vi "Puzzle 1-1.vi"() -> ()   [LabVIEW 2022 SP3]
panel:
  out "sum":i32=54450
  out "Array 3":i32[](array[numeric])=[11, 53, 81, 79, 28, 61, 81, 25, 44, 61, 17, 88, 22, 94, 45, 76, 32, 22, 13, 88, 17, 66, 11, 75, 55, 22, 75, 77, 79, 45, 55, 81, 33, 89, 76, 24, 73, 86, 22, 71, 99, 15, 66, 11, 11, 26, 99, 97, 77, 82, 33, 52, 95, 44, 22, 28, 34, 44, 28, 18, 77, 61, 86, 32, 66, 99, 66, 32, 91, 55, 43, 44, 12, 41, 96, 25, 77, 11, 27, 87, 88, 43, 16, 27, 55, 44, 22, 55, 71, 97, 83, 79, 99, 62, 27, 11, 88, 11, 66, 45, 63, 53, 33, 41, 35, 53, 92, 44, 22, 19, 65, 44, 11, 78, 58, 13, 13, 47, 11, 77, 55, 66, 32, 22, 11, 22, 54, 44, 96, 13, 59, 71, 22, 88, 29, 58, 33, 98, 43, 65, 11, 44, 66, 33, 74, 58, 41, 66, 38, 11, 81, 44, 99, 99, 83, 99, 33, 67, 75, 33, 75, 33, 55, 22, 88, 22, 29, 69, 33, 18, 39, 11, 36, 22, 98, 34, 32, 54, 48, 71, 56, 88, 51, 18, 11, 71, 77, 33, 55, 77, 21, 16, 14, 21, 16, 69, 88, 49, 31, 98, 85, 33, 14, 66, 62, 91, 88, 62, 68, 22, 14, 24, 94, 62, 58, 62, 19, 41, 67, 61, 59, 77, 92, 38, 77, 72, 95, 77, 35, 45, 33, 89, 77, 77, 31, 13, 46, 48, 77, 33, 71, 55, 85, 11, 63, 77, 55, 83, 88, 87, 44, 34, 33, 97, 55, 99, 55, 77, 27, 21, 22, 66, 55, 28, 42, 33, 84, 82, 64, 21, 78, 55, 58, 82, 34, 13, 62, 53, 28, 22, 94, 22, 85, 88, 47, 31, 88, 32, 33, 77, 47, 57, 21, 17, 54, 77, 32, 11, 66, 71, 93, 33, 49, 66, 11, 83, 23, 99, 27, 11, 85, 95, 85, 46, 12, 38, 86, 13, 52, 66, 78, 82, 77, 77, 11, 44, 99, 89, 88, 31, 55, 44, 42, 75, 66, 42, 19, 88, 58, 78, 77, 32, 15, 44, 77, 76, 85, 28, 93, 37, 42, 22, 11, 14, 22, 82, 86, 77, 93, 99, 44, 54, 99, 22, 88, 55, 17, 11, 61, 13, 57, 39, 66, 55, 27, 94, 41, 49, 66, 61, 11, 22, 99, 27, 55, 24, 34, 73, 95, 72, 59, 88, 24, 24, 98, 63, 29, 77, 55, 39, 99, 89, 16, 38, 92, 37, 98, 66, 99, 57, 27, 23, 44, 47, 88, 79, 33, 55, 88, 11, 99, 77, 32, 66, 77, 64, 57, 99, 69, 44, 63, 56, 55, 99, 33, 66, 44, 17, 43, 98, 74, 24, 11, 93, 33, 23, 41, 99, 74, 64, 85, 91, 57, 77, 88, 79, 49, 33, 44, 33, 91, 29, 17, 51, 64, 82, 75, 53, 11, 21, 51, 33, 46, 91, 55, 22, 98, 59, 66, 66, 44, 14, 55, 44, 61, 29, 39, 91, 66, 76, 78, 97, 52, 44, 53, 17, 35, 26, 33, 55, 44, 77, 24, 97, 44, 33, 94, 43, 99, 47, 24, 44, 72, 63, 44, 72, 12, 55, 88, 42, 28, 44, 67, 47, 33, 68, 95, 75, 66, 92, 34, 77, 54, 84, 66, 74, 29, 25, 81, 18, 11, 98, 24, 32, 29, 88, 35, 88, 34, 33, 55, 61, 41, 11, 33, 45, 39, 86, 77, 77, 77, 23, 87, 89, 77, 77, 55, 98, 56, 22, 92, 99, 87, 66, 35, 33, 15, 88, 11, 25, 13, 47, 23, 52, 86, 99, 68, 33, 44, 99, 87, 11, 77, 22, 81, 27, 48, 83, 22, 22, 72, 77, 33, 56, 18, 59, 44, 11, 11, 15, 77, 33, 84, 87, 73, 99, 88, 48, 43, 88, 37, 52, 91, 95, 77, 57, 67, 44, 84, 33, 99, 34, 44, 33, 66, 75, 61, 67, 84, 26, 52, 11, 55, 99, 48, 37, 55, 71, 44, 68, 19, 33, 94, 29, 81, 22, 92, 44, 21, 87, 66, 66, 22, 33, 68, 85, 44, 85, 44, 68, 37, 15, 22, 31, 44, 61, 53, 34, 45, 86, 36, 55, 48, 96, 88, 94, 85, 55, 41, 44, 47, 22, 33, 44, 29, 44, 54, 97, 18, 44, 76, 36, 43, 83, 99, 99, 71, 73, 41, 85, 88, 99, 59, 26, 47, 98, 28, 72, 44, 11, 11, 52, 44, 32, 25, 96, 18, 33, 56, 55, 44, 98, 61, 77, 11, 45, 94, 16, 65, 79, 88, 62, 77, 55, 61, 28, 99, 31, 67, 27, 78, 35, 66, 99, 42, 22, 77, 66, 37, 27, 22, 49, 66, 94, 54, 84, 14, 51, 29, 44, 91, 45, 46, 19, 18, 88, 22, 46, 92, 85, 89, 75, 27, 11, 33, 56, 77, 22, 75, 15, 53, 25, 33, 58, 16, 59, 36, 45, 42, 64, 59, 44, 66, 33, 34, 59, 38, 56, 66, 75, 22, 24, 27, 27, 11, 26, 22, 42, 22, 28, 99, 98, 44, 78, 66, 65, 19, 59, 28, 77, 98, 92, 65, 11, 16, 22, 66, 66, 38, 79, 75, 99, 11, 15, 66, 95, 22, 88, 14, 22, 52, 82, 22, 46, 83, 66, 77, 81, 22, 83, 58, 68, 55, 38, 26, 54, 55, 33, 53, 11, 33, 85, 81, 95, 32, 74, 99, 71, 23, 11, 25, 74, 94, 88, 23, 39, 53, 11, 13, 96, 44, 88, 54, 26, 66, 77, 33, 99, 54, 17, 85, 77, 23, 66, 54, 97, 55, 78, 36, 33, 27, 69, 16, 49, 66, 62, 76, 88, 86, 65, 45, 24, 44, 68, 33, 46, 33, 96, 96, 22, 44, 86, 77, 52, 66, 83, 55, 64, 11, 55, 69, 33, 88, 55, 55, 19, 95, 94, 46, 31, 88, 32, 77, 48, 22, 49, 77, 96, 49, 55, 33, 81, 98, 33, 33, 24, 97, 55, 45, 77, 48, 11, 77, 44, 44, 69, 43, 67, 99, 58, 76, 66, 42, 88, 46, 55, 88, 66, 99, 51, 42, 65, 47, 82, 59, 43, 22, 87, 77, 29]
  out "Array 2":string[](array[string])=["1", "5", "8", "7", "2", "6", "8", "2", "4", "6", "1", "8", "2", "9", "4", "7", "3", "2", "1", "8", "1", "6", "1", "7", "5", "2", "7", "7", "7", "4", "5", "8", "3", "8", "7", "2", "7", "8", "2", "7", "9", "1", "6", "1", "1", "2", "9", "9", "7", "8", "3", "5", "9", "4", "2", "2", "3", "4", "2", "1", "7", "6", "8", "3", "6", "9", "6", "3", "9", "5", "4", "4", "1", "4", "9", "2", "7", "1", "2", "8", "8", "4", "1", "2", "5", "4", "2", "5", "7", "9", "8", "7", "9", "6", "2", "1", "8", "1", "6", "4", "6", "5", "3", "4", "3", "5", "9", "4", "2", "1", "6", "4", "1", "7", "5", "1", "1", "4", "1", "7", "5", "6", "3", "2", "1", "2", "5", "4", "9", "1", "5", "7", "2", "8", "2", "5", "3", "9", "4", "6", "1", "4", "6", "3", "7", "5", "4", "6", "3", "1", "8", "4", "9", "9", "8", "9", "3", "6", "7", "3", "7", "3", "5", "2", "8", "2", "2", "6", "3", "1", "3", "1", "3", "2", "9", "3", "3", "5", "4", "7", "5", "8", "5", "1", "1", "7", "7", "3", "5", "7", "2", "1", "1", "2", "1", "6", "8", "4", "3", "9", "8", "3", "1", "6", "6", "9", "8", "6", "6", "2", "1", "2", "9", "6", "5", "6", "1", "4", "6", "6", "5", "7", "9", "3", "7", "7", "9", "7", "3", "4", "3", "8", "7", "7", "3", "1", "4", "4", "7", "3", "7", "5", "8", "1", "6", "7", "5", "8", "8", "8", "4", "3", "3", "9", "5", "9", "5", "7", "2", "2", "2", "6", "5", "2", "4", "3", "8", "8", "6", "2", "7", "5", "5", "8", "3", "1", "6", "5", "2", "2", "9", "2", "8", "8", "4", "3", "8", "3", "3", "7", "4", "5", "2", "1", "5", "7", "3", "1", "6", "7", "9", "3", "4", "6", "1", "8", "2", "9", "2", "1", "8", "9", "8", "4", "1", "3", "8", "1", "5", "6", "7", "8", "7", "7", "1", "4", "9", "8", "8", "3", "5", "4", "4", "7", "6", "4", "1", "8", "5", "7", "7", "3", "1", "4", "7", "7", "8", "2", "9", "3", "4", "2", "1", "1", "2", "8", "8", "7", "9", "9", "4", "5", "9", "2", "8", "5", "1", "1", "6", "1", "5", "3", "6", "5", "2", "9", "4", "4", "6", "6", "1", "2", "9", "2", "5", "2", "3", "7", "9", "7", "5", "8", "2", "2", "9", "6", "2", "7", "5", "3", "9", "8", "1", "3", "9", "3", "9", "6", "9", "5", "2", "2", "4", "4", "8", "7", "3", "5", "8", "1", "9", "7", "3", "6", "7", "6", "5", "9", "6", "4", "6", "5", "5", "9", "3", "6", "4", "1", "4", "9", "7", "2", "1", "9", "3", "2", "4", "9", "7", "6", "8", "9", "5", "7", "8", "7", "4", "3", "4", "3", "9", "2", "1", "5", "6", "8", "7", "5", "1", "2", "5", "3", "4", "9", "5", "2", "9", "5", "6", "6", "4", "1", "5", "4", "6", "2", "3", "9", "6", "7", "7", "9", "5", "4", "5", "1", "3", "2", "3", "5", "4", "7", "2", "9", "4", "3", "9", "4", "9", "4", "2", "4", "7", "6", "4", "7", "1", "5", "8", "4", "2", "4", "6", "4", "3", "6", "9", "7", "6", "9", "3", "7", "5", "8", "6", "7", "2", "2", "8", "1", "1", "9", "2", "3", "2", "8", "3", "8", "3", "3", "5", "6", "4", "1", "3", "4", "3", "8", "7", "7", "7", "2", "8", "8", "7", "7", "5", "9", "5", "2", "9", "9", "8", "6", "3", "3", "1", "8", "1", "2", "1", "4", "2", "5", "8", "9", "6", "3", "4", "9", "8", "1", "7", "2", "8", "2", "4", "8", "2", "2", "7", "7", "3", "5", "1", "5", "4", "1", "1", "1", "7", "3", "8", "8", "7", "9", "8", "4", "4", "8", "3", "5", "9", "9", "7", "5", "6", "4", "8", "3", "9", "3", "4", "3", "6", "7", "6", "6", "8", "2", "5", "1", "5", "9", "4", "3", "5", "7", "4", "6", "1", "3", "9", "2", "8", "2", "9", "4", "2", "8", "6", "6", "2", "3", "6", "8", "4", "8", "4", "6", "3", "1", "2", "3", "4", "6", "5", "3", "4", "8", "3", "5", "4", "9", "8", "9", "8", "5", "4", "4", "4", "2", "3", "4", "2", "4", "5", "9", "1", "4", "7", "3", "4", "8", "9", "9", "7", "7", "4", "8", "8", "9", "5", "2", "4", "9", "2", "7", "4", "1", "1", "5", "4", "3", "2", "9", "1", "3", "5", "5", "4", "9", "6", "7", "1", "4", "9", "1", "6", "7", "8", "6", "7", "5", "6", "2", "9", "3", "6", "2", "7", "3", "6", "9", "4", "2", "7", "6", "3", "2", "2", "4", "6", "9", "5", "8", "1", "5", "2", "4", "9", "4", "4", "1", "1", "8", "2", "4", "9", "8", "8", "7", "2", "1", "3", "5", "7", "2", "7", "1", "5", "2", "3", "5", "1", "5", "3", "4", "4", "6", "5", "4", "6", "3", "3", "5", "3", "5", "6", "7", "2", "2", "2", "2", "1", "2", "2", "4", "2", "2", "9", "9", "4", "7", "6", "6", "1", "5", "2", "7", "9", "9", "6", "1", "1", "2", "6", "6", "3", "7", "7", "9", "1", "1", "6", "9", "2", "8", "1", "2", "5", "8", "2", "4", "8", "6", "7", "8", "2", "8", "5", "6", "5", "3", "2", "5", "5", "3", "5", "1", "3", "8", "8", "9", "3", "7", "9", "7", "2", "1", "2", "7", "9", "8", "2", "3", "5", "1", "1", "9", "4", "8", "5", "2", "6", "7", "3", "9", "5", "1", "8", "7", "2", "6", "5", "9", "5", "7", "3", "3", "2", "6", "1", "4", "6", "6", "7", "8", "8", "6", "4", "2", "4", "6", "3", "4", "3", "9", "9", "2", "4", "8", "7", "5", "6", "8", "5", "6", "1", "5", "6", "3", "8", "5", "5", "1", "9", "9", "4", "3", "8", "3", "7", "4", "2", "4", "7", "9", "4", "5", "3", "8", "9", "3", "3", "2", "9", "5", "4", "7", "4", "1", "7", "4", "4", "6", "4", "6", "9", "5", "7", "6", "4", "8", "4", "5", "8", "6", "9", "5", "4", "6", "4", "8", "5", "4", "2", "8", "7", "2"]
  out "Array":string[](array[string])=["1", "3", "1", "9", "8", "1", "1", "5", "4", "1", "7", "8", "2", "4", "5", "6", "2", "2", "3", "8", "7", "6", "1", "5", "5", "2", "5", "7", "9", "5", "5", "1", "3", "9", "6", "4", "3", "6", "2", "1", "9", "5", "6", "1", "1", "6", "9", "7", "7", "2", "3", "2", "5", "4", "2", "8", "4", "4", "8", "8", "7", "1", "6", "2", "6", "9", "6", "2", "1", "5", "3", "4", "2", "1", "6", "5", "7", "1", "7", "7", "8", "3", "6", "7", "5", "4", "2", "5", "1", "7", "3", "9", "9", "2", "7", "1", "8", "1", "6", "5", "3", "3", "3", "1", "5", "3", "2", "4", "2", "9", "5", "4", "1", "8", "8", "3", "3", "7", "1", "7", "5", "6", "2", "2", "1", "2", "4", "4", "6", "3", "9", "1", "2", "8", "9", "8", "3", "8", "3", "5", "1", "4", "6", "3", "4", "8", "1", "6", "8", "1", "1", "4", "9", "9", "3", "9", "3", "7", "5", "3", "5", "3", "5", "2", "8", "2", "9", "9", "3", "8", "9", "1", "6", "2", "8", "4", "2", "4", "8", "1", "6", "8", "1", "8", "1", "1", "7", "3", "5", "7", "1", "6", "4", "1", "6", "9", "8", "9", "1", "8", "5", "3", "4", "6", "2", "1", "8", "2", "8", "2", "4", "4", "4", "2", "8", "2", "9", "1", "7", "1", "9", "7", "2", "8", "7", "2", "5", "7", "5", "5", "3", "9", "7", "7", "1", "3", "6", "8", "7", "3", "1", "5", "5", "1", "3", "7", "5", "3", "8", "7", "4", "4", "3", "7", "5", "9", "5", "7", "7", "1", "2", "6", "5", "8", "2", "3", "4", "2", "4", "1", "8", "5", "8", "2", "4", "3", "2", "3", "8", "2", "4", "2", "5", "8", "7", "1", "8", "2", "3", "7", "7", "7", "1", "7", "4", "7", "2", "1", "6", "1", "3", "3", "9", "6", "1", "3", "3", "9", "7", "1", "5", "5", "5", "6", "2", "8", "6", "3", "2", "6", "8", "2", "7", "7", "1", "4", "9", "9", "8", "1", "5", "4", "2", "5", "6", "2", "9", "8", "8", "8", "7", "2", "5", "4", "7", "6", "5", "8", "3", "7", "2", "2", "1", "4", "2", "2", "6", "7", "3", "9", "4", "4", "9", "2", "8", "5", "7", "1", "1", "3", "7", "9", "6", "5", "7", "4", "1", "9", "6", "1", "1", "2", "9", "7", "5", "4", "4", "3", "5", "2", "9", "8", "4", "4", "8", "3", "9", "7", "5", "9", "9", "9", "6", "8", "2", "7", "8", "6", "9", "7", "7", "3", "4", "7", "8", "9", "3", "5", "8", "1", "9", "7", "2", "6", "7", "4", "7", "9", "9", "4", "3", "6", "5", "9", "3", "6", "4", "7", "3", "8", "4", "4", "1", "3", "3", "3", "1", "9", "4", "4", "5", "1", "7", "7", "8", "9", "9", "3", "4", "3", "1", "9", "7", "1", "4", "2", "5", "3", "1", "1", "1", "3", "6", "1", "5", "2", "8", "9", "6", "6", "4", "4", "5", "4", "1", "9", "9", "1", "6", "6", "8", "7", "2", "4", "3", "7", "5", "6", "3", "5", "4", "7", "4", "7", "4", "3", "4", "3", "9", "7", "4", "4", "2", "3", "4", "2", "2", "5", "8", "2", "8", "4", "7", "7", "3", "8", "5", "5", "6", "2", "4", "7", "4", "4", "6", "4", "9", "5", "1", "8", "1", "8", "4", "2", "9", "8", "5", "8", "4", "3", "5", "1", "1", "1", "3", "5", "9", "6", "7", "7", "7", "3", "7", "9", "7", "7", "5", "8", "6", "2", "2", "9", "7", "6", "5", "3", "5", "8", "1", "5", "3", "7", "3", "2", "6", "9", "8", "3", "4", "9", "7", "1", "7", "2", "1", "7", "8", "3", "2", "2", "2", "7", "3", "6", "8", "9", "4", "1", "1", "5", "7", "3", "4", "7", "3", "9", "8", "8", "3", "8", "7", "2", "1", "5", "7", "7", "7", "4", "4", "3", "9", "4", "4", "3", "6", "5", "1", "7", "4", "6", "2", "1", "5", "9", "8", "7", "5", "1", "4", "8", "9", "3", "4", "9", "1", "2", "2", "4", "1", "7", "6", "6", "2", "3", "8", "5", "4", "5", "4", "8", "7", "5", "2", "1", "4", "1", "3", "4", "5", "6", "6", "5", "8", "6", "8", "4", "5", "5", "1", "4", "7", "2", "3", "4", "9", "4", "4", "7", "8", "4", "6", "6", "3", "3", "9", "9", "1", "3", "1", "5", "8", "9", "9", "6", "7", "8", "8", "2", "4", "1", "1", "2", "4", "2", "5", "6", "8", "3", "6", "5", "4", "8", "1", "7", "1", "5", "4", "6", "5", "9", "8", "2", "7", "5", "1", "8", "9", "1", "7", "7", "8", "5", "6", "9", "2", "2", "7", "6", "7", "7", "2", "9", "6", "4", "4", "4", "4", "1", "9", "4", "1", "5", "6", "9", "8", "8", "2", "6", "2", "5", "9", "5", "7", "1", "3", "6", "7", "2", "5", "5", "3", "5", "3", "8", "6", "9", "6", "5", "2", "4", "9", "4", "6", "3", "4", "9", "8", "6", "6", "5", "2", "4", "7", "7", "1", "6", "2", "2", "2", "8", "9", "8", "4", "8", "6", "5", "9", "9", "8", "7", "8", "2", "5", "1", "6", "2", "6", "6", "8", "9", "5", "9", "1", "5", "6", "5", "2", "8", "4", "2", "2", "2", "2", "6", "3", "6", "7", "1", "2", "3", "8", "8", "5", "8", "6", "4", "5", "3", "3", "1", "3", "5", "1", "5", "2", "4", "9", "1", "3", "1", "5", "4", "4", "8", "3", "9", "3", "1", "3", "6", "4", "8", "4", "6", "6", "7", "3", "9", "4", "7", "5", "7", "3", "6", "4", "7", "5", "8", "6", "3", "7", "9", "6", "9", "6", "2", "6", "8", "6", "5", "5", "4", "4", "8", "3", "6", "3", "6", "6", "2", "4", "6", "7", "2", "6", "3", "5", "4", "1", "5", "9", "3", "8", "5", "5", "9", "5", "4", "6", "1", "8", "2", "7", "8", "2", "9", "7", "6", "9", "5", "3", "1", "8", "3", "3", "4", "7", "5", "5", "7", "8", "1", "7", "4", "4", "9", "3", "7", "9", "8", "6", "6", "2", "8", "6", "5", "8", "6", "9", "1", "2", "5", "7", "2", "9", "3", "2", "7", "7", "9"]
  out "subarray":string[](array[string])=["ninefourone1", "53sevenvvqm", "kscpjfdxp895foureightckjjl1", "72fivebt9ndgq", "28gtbkszmrtmnineoneightmx", "four66jqrbtqcsxjtqjvfjhl1", "four8pzznjbhxlhtz6bhtzdxjlg1", "rgxjrsldrfmzq25szhbldzqhrhbjpkbjlsevenseven", "slkjvk4threesevenznjqmmfive", "61ppgrkmkfhteightone", "1threesix67px", "sxbjdbtlnjrmlzgxneightthreepmqxdxhfk8jfrheightwovp", "twofour2sevenk", "sevenonezknqnkfqbzffjvfivetwo94two", "45xj", "mp7one6eightvhfnmfive6", "fhtctftxm3threefour2b", "2dq7bdmhhs92", "pdnbqlbvtcxgpnfhmsfhzstgm173", "8fourvxkddsrlcvseveneight", "15zqpmsix77hlljgfive", "jzjv6seven", "eight1vbfive", "721sixsdzbqtskbpkqbcmgmlpk5psrhr", "pqxdxcx5", "twozsf2five", "7twosixthree775", "7xtxrch7six", "729twofourlqrxtwo", "qtvbgtclhnk4ninefourseven5one", "jvhngkcdjhnmqghdbqdzqssf5onegzjbbcchboneightn", "five8two14five2nine1", "one3twomddthree", "8nine9two", "7fiveeight9ninesix6fivethree", "254kcd61dc4two", "7sixonetxvthntlngtwobzkbz23", "8sixnine6", "threedqtgmv2skmvcd", "7ptdhpvr1", "lsvmzvzvd9mqxszjmbddkmxzdxsninedmglzlzphtwo", "kgdt12seven4xxtttr5", "nrdtgdftjmfour6fxjninenineblqlthvpcx", "ninezmstcdfchc11onebmmfdfhvdncrhc", "1fiveseven", "oneone26twoeight", "threefivenine98one9twotbbcq", "9cm7ninestc", "jcrbmcjtrlzvz7", "nine8nine22", "3nineoneseveneight", "58four2three", "stwonefourthree9twonine4six5bvxgkxf", "ninechzcz4seven", "2tgzgmtzzpjdqqz", "brsptjppb28qxcxxjbzpeighteight", "eightthree3ninejrft4", "sixqsgkzdjmgpfive4threemxltqdxsfive", "vxfd2q8", "khqhgqlxslkmbrvljcnineeight1gjgcqmnbdczqb8four", "mvbltrgpfourcclxftbb7gcbqcptvgfsevenrdm", "61eight", "six8fourthree6fourseven6three", "jqdfxvhjg3sflkn2sixptxxsqrfml", "6jtxs", "seven99threeone", "five6sevensmbbrjqvdbmkbsqtwonelg", "fdvfsndt32fourgllgfrninebhnzzczfive", "9hxp9srhjhjjvqljhzprcjpqreightzs1", "djldhkkcn55threethreefourflnxnbzhkzmx", "fourfive43chfvjnvjrkpxlgjrfnqbl", "fxjgtj4", "1sevenfour2fiveeight", "seven43rxxeightb1", "9sevensnxkp3lpzxfxnntkxzkrhk7jzhmtvn6", "25one", "threeone7", "1pkfvsxxthreeoneseven", "ztbvfqnpz2xdhgdjmgvfourtworqbxqsh47", "8four7sixninesix", "threedgl88cczqhqxjnc", "nineeightthree4sixfive3sixdqlmscqjk", "16crjsdl", "tgq2sixhc7three", "tzgsqspndt5xnqlthghzfvkkhone", "4fxdqrs64ninex34gd", "seven22", "kghfkrpvnppfncbhhqpt55bjf", "hjhb71bqdrrgsrkqdtsgrxgsscqjmtfzjkzsbp", "lgdnt9threeeighteight97", "pvjhnk83sixncvgmsjltwotdmmpxknhvntfndxr", "7449", "qdfzv9hkprplzkfh", "66three5five4zdsfrcnljqmsxf2", "veightwo27bdbsvseveneightrcqcjxsixeight", "1thvkkk", "8bnxqfsdhzppblzlzbkfsksfscmb", "zseventbdzlmhnnrfive1one", "sixxnmntrmp6srcsqbrqnjfiveeightfive", "4trnzlshnjtwo5twocxrvfssbj", "6two3twonetqt", "55qsnx43", "3three23tpctbkrnqv", "sixqk4cnfdmtltmlhqxtwo41glkhdhgnt", "35fivesevenpfournxzsbbgzthjvlvzrnine", "tworkzgkcvcone53nrvgdvgtc", "two9llkjbkz8pklrsgqqzr2four", "ninecgpbgcnine4tldjqsone4six", "2tfjhtfourfour", "onebhlhdvvqx1sevenmsixsix9", "pjgjt6jkrgshxltfnine8four45", "4vsqfljrfiveqeightnvbdb", "11nfslqvhm", "7crrhqxsfive8ctkzbhqnine", "vrvtglvthreettrkq5bdlrtpx718", "1btbxlthreedtrzgeightnineqczhqm3", "193", "fcbzxqxxjtmn47ffschdrbeight", "twoh1gqkrnm1", "7ninesixpzpsn7", "5kkvzpgqd", "three6nine", "32fdn", "22twoxgvktxpxmbjqtgtbckx", "1hdtftwosix", "2jfc", "six5nvzcgmrscjn5eight4", "nineqhtczsninetwosix4five", "9three6sj", "hntktlbqmldrphqzxkhfour193", "twotwo5259", "v7six1vtlxnpm", "rhsm2", "gprmtxbhlsv8onefournine", "2fsrbtdvft15six1kxpqbnqsxh9", "one5onemxthree8", "nineqbxdbznzktxsmstsntzffour3one", "9blhkhjsgsfgsblzdtqqfour8", "stz4889563cb", "vjrbs6threeptbbmncz7hqhqgfgldtseven5", "vbfs1", "zjqgczjsjpvzvjseven4", "sixfjzbrrhcfqvglxhnsxninedrvtvjbfqjdbrzblkq6three", "one3threegcdldjsrsssixonefiveonechngsl", "7srxv4hsgjqsqfvv1tdngkpjrczkl4", "5scgdglnjbnsix8fivesixtjccvmkfxfnzvhctgpncjc", "4eightfivefive1lgscbj7kpcr1", "eightknfssevenfive6jnpklczrpfeightwol", "37qccxllhzshninebvpc8", "1eightmmcthkhf", "seven8fourqn7tbgqnmzcc1", "sixsevenone4", "clhdvjnqnine9threesix", "onetwoeight9", "81z3threenjsdhnqxvtwonezv", "9hqtsb", "onekgnlbthreeg3", "eightspnrpjb65fivevzfpvjntbg7drbgjccneight", "ninerdlsix7285", "fournineninefive3vbnhmhdvjgdqcm", "njzspqxpxrone7four55", "nfdhlqcpvzrrtsmzhgq3", "fourmfdtnpsfbxkjtgtgx5sixrppsqplqdjvnsixdtqvtdm", "21onesix6sixnine2", "fffsmvtt8fivenineglrqrmktzzseven", "fivefoursevencjxmskrqclz2", "lgk27threefourfsqrbkntbkfourvflgrzhh9", "617hj9", "ninegcxninetwohpfdxrb3tjjjtxtnvtwo", "one1gnftc8onehtsxsmg", "foneight3fsbhdqzr5twojbsdnntwohd9seven", "zkzpfvcxqnbvrg1", "nine36cddqfvrf", "rdjlpfk2pschfsdrpz", "nine994three8six", "three3nvflpftf2eight4", "3nine2", "rxxjdk5354", "hf4eight8qjtcfldnkvtwofivetwothree", "7six3twodhnvmxj1nine", "57seven3six6", "qklbvzfhclfnllhhgeight8xtvld", "5fgzqhkssmkcfour1", "hhvjkdnlffnineeighttwo18twonecs", "sevenbfzrgfm1six1", "nine71cskklxvcbnxtskdbqnpgklrxklcgccxjnssksrlkx", "hmklhhjdthree77", "3vpxclbgkpone3ninesrclfive", "djfqkgjvqpfvdsix5sixtwoeightsix", "eightlt7csvgxpnslk", "sevenfoureightnld2mxtgpbzpthree1", "11sevenglfmsb6", "onetjjnxvssg1four4drxbxpnpv24", "2zdxs9mfnbgfmjln1threefive", "one186ltsbck", "6fsbpb9sixhc", "nine818", "xzqcpcdprsqjbgknkvztwo419q", "39qfdlcnkhg31", "9djnlcrxqxhrcb8mczrxrm", "nmb887525seven", "jhmv3", "zhvdbn1fivem8seven4sixoneighttsn", "6zmmjqmnftclqbcthree", "6cpzeight92", "onepqfhtsevencvlfvnczhb91mmtdprqxmcnine1", "tvqdfxn8eight", "five6fivercgrpbtjgv87jmcndclbk2six", "jgtmrbvl68lpqkpxddqqxvsixfivesix", "nine2nlffgkvmp", "1frdnhssftg4eightgclxsgqtn", "2sixblr94six", "94mlfv", "6vlqtcsmdd47hpfmlc7fiveeight2", "tklxghxv5bzc4hhcdcpmnine8", "four6one1zzgqghvs412", "xghjpblsfpg19ntpfmcfd", "471rbdblzs", "69fourhjxkvd7fourfour", "jmrscfqdfppfdjskpk61", "five5eightnqpd9ninezknztwo", "onelknchr7nrfprgmqzp", "svxlxrx9892five2", "3ntkbzzpxhdmrsix8ttgp", "ndh7zlnrzpvmnine", "one7xlnbmjjmfv62qvqjpfprbvjkpcnine", "99three5", "threetwotwo7dhtgtbchc7sixtwo", "tmfxxph3eightgdccscdsrkmnhbb75", "joneight4one5", "nine3six", "81tqzsqpkv99", "sixvjlq7", "five7bkc", "five3811threelfpzztxzk", "1fourkkpclqc3", "xgrpbmktcthree46g", "bgcp4two8", "jtgeightwo7nine", "bkmcrcq3eightrdtvrbglmxmmztqm", "7tscmg5one2jhhbfb1", "zt5khcrgqjg5nxxzxzd", "five85", "twothree1", "eightsixthreetwo6b3tnjmcqdjfive", "onefrlg7", "fivescbjxbdnvslqqsone5bdbvskpmksqmmfsncsmd", "two83fourthreefourseventhree", "dglrmbtkfltwofive8ninelzmrxvxoneeight", "8nine6sixsixtwo7", "sevennine4lbsevenkdnrhpltn", "h3fiveeight4cplrnd", "vhsgjbqm3ninedfhfsb", "93nine7jvjmlzgcztrqlxtwo", "zhhhdddbbgcssvfzdhmpone5fivefournine", "l9fourvjfbqpdslkmvxsdrnsgcvzpjxm", "kxlseven5two", "rbtwonegsdgvsjtpnnkone7mdz", "phffknvthree2threeqgvfqxgnine7", "2lgglnmthreeseven27three81", "lrgkrxx2", "seventwokxvzkvq6eightthree", "5fiveseven", "fstwonersngdlngx28nine", "49oneninesix8four2q", "hfvhzvmjgbfcbsevenrmhjhzkc3", "six84", "8eight2gzblldzvkjfive", "6fz3eightzmsqb4qsbbsnthm", "fcglpc2one51", "sevendqghclrpxt7pzone48two", "three5one", "5sevenfivebbzkjlcnxseven8fourmzqlxxgjvc", "xgg8one6782", "gggtljnnsix3lkhdqzzpdtdkmjtgjddkpgx4five", "qrmsfc13onevnhlbgs", "nrtwonethreerbbqffzh62", "5eight81gcdbrx3rlk", "mtdtxcmm2bgmqhgqrtxsn8", "onercx2", "9sixoneqgr4", "xmoneightfour2", "six85foursixninetwo", "ninetwo8four8six", "qchclfzq47", "khrll3two21", "seveneightnine8868four", "3rmbmtbxjp12seven", "3tsxgvqxmzvxbdvxtgrvdbzqbh", "eight7fourjtxx", "fmb4one7threekbxeightwoj", "vcsevensixseven577", "2dkhlrrtrnbgzrmxm5fiveclhgn1eight", "1sevenlmrbnfour17seven", "three5jtbvkseightoneseven4df", "fourrgqxplbpbxtsgkm7", "fourqdfxchlc371sc2", "fqxlmeighttwo1seven", "zvvlftlhfthreesix6three46qkstxvdt", "m74pjgccfour1four", "plphq933eighteight", "cdbqlhbhj3eight", "4onevgdkxhz799five9fbljhpqmvk", "two6qzgphxl", "two1eight", "onekxxghlonerqqlrs83threehvvdhsxmfour", "npmsvvrdl2673", "fivejthseightsixtwo9vgrvjzbzsrxjv", "eight2gqfive7mzjzpxqcvheightjfx", "1bxckdpt", "dngoneightbtdptfn85", "fourtwovfzgmxjseven935", "8onesix2drgjnlrxbtdlmlznine5", "five4mmpmqlttsx56ljdzldntdvthree", "1nxxgtwothree22twothreenine", "38eightsevennxctjfstp", "8fourvhnps3onellstpnztn6kvjccmv", "1bseven93eightfour", "5nphkdbhxqb2pqxtkvhxq", "nvvx6fourjgkdsczjv", "fourxrmq78", "8tjmnvthree3ninetwo2five", "p7cvtwoneq", "7thbggjbznrsixonethreeninej", "xdgm1crqfnklk", "onehmqqgh4ninenthjonegfjmvtfgd", "sevenbsqtlk9", "8seven9two9hdz29", "fbcjhzdgzdg8jgjvcrmgbcrsixnine", "3bssqrj44onedqxvhkfive1", "tmmxtz5dtxbbcjlfivesix", "pvfqzksgrs4khmlvtwoeightlsx", "psbttsmnpninefour42fivegsixfive", "sevenfiveqscr7dfxpninesix5", "xmsjddzfxftsjfq6four6eight6three", "seven42", "eighteight1nineeight9", "8c", "pmqljjjzvx5znxqnsfour8", "78zlpxnvsqpgmgmk", "four7fsgttnrgnlslr", "fourtwo3jg2", "qlz18three5lpxfjvnfppqjxh", "4fiveonetthree4eight", "7lzffxkxnzjrtr", "three7nineone46ksnshqgdpt", "8dntxkkkgdxggvhxh2onefour5gqzsqkm", "tjsixonedbklrxxk2twonxdpjzb8", "mfglbrjrq93", "seven37xhsrxrvcgninexbmdrzxthreeonethree", "fivegznvfztszqlhtrsslsmqq43212", "tdthjjjbkeighteightsevenpcbmpfq2", "five1eightq", "three13three4vrsrrtp", "cgztjgqgdths2", "dhxztfvlonetwokszrv8prdpm2", "dfkcklchjj8twonine52ppvndfcnf6", "three7ninenkxfourfive", "93sixlqxctdhmvssixone", "oneqbvfrvteightnineninefivethree9", "jskrtmvsrqnpvcgsmxbonecmlrjpdpc4three", "crpcfour54xxgzz", "9fivefhdpcqsd", "fivenineclfctjninefbsh2", "fivexhrzbqpfxl8sixtwoeightllzplcpllk", "zxgl5qneightsevenone", "sixpdc17thxfive", "1twolftpzbmnzvdlkvlsevenhdvgfrjhmthreethreeddkdvht", "67twotwo71", "oneeightcgnhtdxpfnsevenoneeight13", "eightthreervd5tnj17", "ssrsmhxrsixeight3gbqggcvfqg29", "6fivecvcdxnxhxxtlzthree", "fournrrsix595", "p2qchlvplzdvchkbdzzbnsix7ninefour", "fourthreefourtzvlrnr9m94seven", "4jxzkrfourvtjpsnrllkjcczmmqnsj4q1two", "4627qlpscgpjcnine539", "two6nineeight", "63five66fivethree1", "skndgzsbsntwoone1", "threerzgdxgtthree2three", "953lsdgn59", "27bk", "sixmfmbslpjjsixsvnqrvtxznffive5", "2ninenlgpggxm42six234", "fdzfvkjnchsevenfivethreetscllgjvrtqckfnmz3cszmt4", "7ninetlzsxjsl2nine3", "shsvptqngsevencjjthvfm9six5four", "7lsrq36threevzfjc62", "two59threedxmfourjfschvqvnine", "khfqjmksxhbvs8sevenhzrmjtkgm", "nine2stgflmsm8fkthhhjzlszdnmkmqpnjxrfc4", "twofourthree244nine", "eightvt978", "fivefiveninesixnine6513", "2lbtz19fourtshqsvblhrkhxbpfour", "ptt7bntxhdvl", "mskflsslvdlmndmmqmfourtczqlssnineseven5xxxkfvzd", "l329eightsevenfourfivethree", "rmlksxsixspp9fourhlcg", "8five9q", "hqoneightsix19nine6xmjbtgjzgrhmlrxq", "six38", "9eight2", "3sixbzhgfcg57sixsixjtqmknd", "9fchn58", "vrpftbnvonefour6", "vqgdtrvhnnxxsevenseven9eight", "56vnine5rdpsnlqcbq7three", "vncrjds2cmrg7", "213sixfivesix", "tzclpzdsthree4sxgjvrzcrzcndnfour", "4sixseven1three7", "8fbrggzmtqn8", "four79p", "twonineqonemfour3dq", "5fdgpmrghtksn5onesixtwo", "xseightwongqqsxtwo8jslclldvnb", "nine1one", "9gxjrfourvhqzcxdhrtpxgtwonine", "eighthfhtnvchtc7fjkrxsmhtm7rbk", "thqxcfjbksix32xqrgqsqtx", "6qjqql", "jgcreight7eight", "6onesix4threeseven", "5vcv1twoeight7", "fivesthreebvjntwo9jdxghmxvl", "632msc9threenineqfone", "dqxfourkb4eight", "6stsp3nine", "566sevenpdmg", "xprjdn55", "9mjtcmhjb", "twoninelkjznqztbc3twolnhjhdbfxmhfr", "twotczpxn6qlcfdlpnq", "4ninefive", "1rs44three2gzczjdgq7ssmtgjbgbb", "ggmzqbkgsix4five23bftjlmbfbd", "threehfcscmmlqvcjtpthree98", "7sixsixone4", "2fivefvrr9four4three", "1zt1seven", "9hsbthqvhhsnineone23tslqccg", "sixbqvd3", "22148four3", "ninejlpbtnfive41rtzqjgfmcbncrrlnn", "9sixfour", "qnhfivetwofjtqtlxd7lmrlfctq864", "69dqrzhlqssgcsxtz54cpmjvrkcfiveseven", "fiveqpv85frkmpgxgc", "xxqsscldeightone9ngqtkf1nine", "5sixgxbnnjsvhf5dgxgone7", "sixsevensqghlvkfxnfour7", "8gmgvjbfivesevennine", "qj796fourone9", "rmpfsppvzdtwo4threetwotwo9", "dqvtrhm3nhtrxxccmfiveonedfzfvcghr", "4threejxkhnxcxjoneightp", "sevenhkpfgdgsgnvseven3m", "qhrvjcnfdbqchrsvchcxfourbkhhq9six1eight", "29pqnd", "1oneonethree627", "5977rcr2threeeight1", "fournthpqbztrhnine64", "fjnjpgqxr86five4sixxhrtvbp2two", "7sdnvlb5two", "58vffgzcgx4nineoneeight3", "h1sjgqbhndbz1oneqgncmhnleightwos", "gjms21", "onetwodphfznine51", "gxpl3fourzfz3", "five46", "mqsixccffmc9gqk1", "5kvxpqrrpeightthree", "threefoursevenfive2dhtbrxlzzl", "shhczssbltllsmntntlqfqgnnl98rm", "5oneeight3vkqtwo29", "bv69fouronefourone6", "eight6five966", "4xnrtztgfgcmnmnsevensix", "gmsvtnjd1sevennine4xxhqfbrjjqbglqjngttc", "mdnxhhteightfive5onenineninegqjbqmfd", "xonefourtwo4", "onesix61", "sjmnjhkj2892eightnine9", "nzseven39", "99nnjjzdrfsnjhthree1sevenfive", "6xmggtbnblnbxdpkzblnvcvjqmhvntwoeightseven", "76five6six", "chdfjrlfhdzeight778", "xrvrck9five1hrvpfvkdcb7eightnine", "foureighttq5sgdfourl2", "4rnbxrhhboneonefournine", "5four3", "1b97eight", "hlcjghlhsf32tgknm565knxqr", "onecqgbgdcmlb2sixsix6nine", "kxdkz3", "seven5xvhrxdm", "xblqbgkqgsixvgrthreezxnzhknklxhbmgl4", "fvnkc7threethreeseven", "bmbqxv24jhdg", "97rfphlxvtx", "4pgblonelone", "ptdpllrddeight3", "9knpjzskrfd4", "twomjqdtbbvmj4shvsqrone3", "9zzh3pjsf6mhxlhm9glglfztjm", "cfconeight47fivetdsmndgvsmbqjvszb", "21vbqjz374", "sixeightqgfdjbhfd4oneeightone", "tbccqdpz78srmcdx4six2", "643gqtvhkljxt", "klfjf4qms", "zrnhkhqzpczzfqsgsrtxklpbtp72", "1cnqfltrmhphg832three", "twoseven5", "mxkmxlcgsixklclrkfr8638fourlrqpzgjq", "nkbfkh452pthree", "zvcktvd2485four88", "rfxj4", "three6jnr7", "two45rldjnmxkjphtwo7v", "fivelncjffdnkzqrshvthreeh3p", "ninejgrbmhrbqldeightnine6nine8one", "96lvpt2djrkc5", "7seveneightthcxgthreeseven5hpfddktpj", "6bvn", "sixbjxtphstzgspnmkcvc952one", "gmmslrndvltlthree394sevenoneightl", "threenine7onefourtwojxhzvqlseveneight", "5eightsix4txcczzmg", "84seven", "skjpkhxggsvjbprhllgjhninetwo6", "72bdpzccvone4zbdzlllnnonernlfvdpq", "bvrtmzmtwonine29", "mrlvmdnlxb2814five5fjxzlhpn", "lmrpf82rksix611", "tvq18oneqnmmzvtclnthree", "jrbjc1zbbpqbrddt26seven1", "lxfivenmdtnhdmf98ptpxsgmgrxkmmznlk", "zbmvchmxsevenddddthree2dxlddjp4", "three3onejg2fqgtjmpcgeighteight", "three2two9seightfjqtwo", "ninefive8sevenvnssix", "3cnbxxtgmf5", "kpmjcsfrjfgzhmbpnqmlvrhbhqs8", "3vvcone64", "fvqksdsixthreexbfivetwo3", "sevenseven5", "63twoone8vhbcpmmlfive1", "4ctwo17eightsixkpvlgpj1", "rsgsnone1", "kbvxonemcqfive3eightone", "ninenineone45threepvsmrtonejxmbnd", "37fklnjkslqk9th9", "fiveoneq8rcgdxtwo8jfkxq6", "rgd7", "7rgkdpvp7qrb", "7crtxfmslxxtcxsv", "mqdnltb23fiveqcdqtonethree", "8seven7", "8cqhqlhndqjznqhdbld2nspnxbj99tqqhp", "onelqn7", "bvbjfour7", "ldqzhvhrbgsrrkh5j", "kjsjxdcqgjztldjvxxgr9twoxfknxrrrphkdzdl8", "rvscnztblp56ljqtwompclcf", "2dbtdgsevenhzctckvkvxvjljz", "tvmhhxbbxvvsnlnineqsltjd92one", "9twoqdmtvbxhpcthreeeight", "81dvnkd87xbct", "6mnxqnndcjfivefdckzmppfsevenmqvvvbnrgs", "lvl3qjk5", "3fivefive", "ktvsqzrf14eightmtnqbcktk5", "sevencdknznbxseventwo8rzggmvpbvlrs", "hkhhrdxlml1xzbshninejzqc", "eightseven23shkgzdgvvcxxfdv5", "14five1sevenxfmhtptwo3seven", "47one", "2three3", "f5dszzs2", "xmxffxkxpkninethree8x6seven", "glzoneighteightrnjqgjznjm9", "63fznqxdfqt8", "33nine", "4vrbmthreefbdzf", "fourninethreesixnine9fourlvbgqhjbqncnlbjbz", "two848dbvbninenine17", "pqzqgone1two", "eight7lmxbhcsix", "szr2fcvkljctlghhthree", "sk81pxqhhhhvnjvgzfiveseven", "cgqqkrz2vpdpzrthqssg7nineeight", "498eightfournine", "eight85onesvxnineone53", "ninevmchpkcg2", "six2shsvqfivefourtwo", "mdzckfvr72cv", "twotwo7onethreefourdjtgjg", "tworfclmm3", "5sfvnkrmrptsix7four6kzlmclm", "1onedkqgzbr89kphvc8", "5seventhree8eight9eight", "kvjpgjgrcmpdscbfthreethree4mjqjnnzceightwohh", "kjbmh1fdkdtznmsznvlconeznineseven", "1fmgpxhxpqznqscvbszhhcmglvtnzhbbjjbzg", "1mfqzkfnine5", "rrflkqslxztdlqxqkdnhqd7ps", "39123thhsmscbpxr", "8vnine4jgqrvqtshg3jhhdnbsrxneight4", "xkqgnfour87", "lsbnjqtzqz7ninenineone73lmkbnkhs", "9fiveqqgqblfivehttxk", "8twotwognd", "4xknbheightfour6358", "4cqtpfjpf72eight3", "ninemjpqpqg8foureightsevenfcvpnrnnpzhcgkm", "37twofivedsxrzbpchnkgxqx", "oneone57one2k92", "mckoneight9threefour1onefourhdrcrvhqcmngkjnsthree", "945", "tmmtwo7", "57", "6twoxzbfftnr27", "threenine4bqpztsixfour", "84eight", "3jpbnjrqhqfnxckqkqdvls", "9gzzjzz", "374nine", "ninembxeight4sevent", "threecq3", "cvn6cvqmpmfflkzphndjnggtktwosn", "pgz7four5nineeightsixqrnfkdkgh", "6one781vstwothreef", "one617fourthreefourxqxnpv", "8eightsqmkjkkf5xckcvd4lfnnfour", "seven23qhntfmg56onexkjxh", "f5s56rfltx282", "twosixninefive1tlzq", "threetdhghclfsksql5oneninetwoseven", "zbqzxmpb9pxlrthree", "r4gxdzjnvzfonejnpmfcpgvxjjvkh8", "five338threejkk67seven", "twolntxcnzvfr55sixtwofivesevennine", "xhlppbqfr71brvppsixthreefddlgpfslqmdv", "kxsklgonefjfpkd4threefive9six4", "6srphqmtdoneh3glthreefour8", "rjzdmj1cqvxnx1nvcvbfctft9", "3fqjdgbpggthreesix53", "9fivesndgmkvckblktzkshglqgdl4ztwoseven", "qqrxkqhnzb23two34nine9", "8hrmffgstqpsixeightx1six", "jngcsjnrhn2zsvcjmjg", "9zfdmhzxdnfour272dcrqgk", "lbjbrfhjxhxjphzxsjsix4", "fourthree2seven1two", "twosix87", "vrlqqkctddggcvcjcpk6hxbqvbxmtsix", "mrcgbpc6dthzqmmthreefour6two", "r2zntjxgpfqfmqh", "fourseven3", "6nfnsgchjdffttmgfnbvlxzoneseven8", "8sevenqqfiveseven5twojvgk", "4rmtkvml4", "bprnine85", "sevenmfpcvlblcnine485fourseven4", "sevenseventhree68fivelhqgjqvcdqkvds", "3fourxsgghqnvtssnvfs7nine7", "1fiveone5hpfdgvxb", "eight2eight42twotwoonenine", "lpdeightxcgpxkkeighthtjpsninemjlxrxtg31", "4smqpjzsixonethree", "mr6csbmgrdrjj3onelqd4four1", "5sixvbscchd3", "384sps", "4qzgsvmfx4ninevcclvcfrfp6tckcpvj5s", "8l5glclltgcjgbhcg6", "3ldtdmjc6threeone", "hsrtzl521nine5qqrtpdsp", "z4v8threejdsmbfjpbj", "9sixln26eightwovmh", "848", "kndxtqpfrqxdxtfnqrqznpgvp9ninerlzcdvdtwo84", "kmqs84775seven", "5threefourzkg", "43five8cq2kprvdqrmxr1", "three4ttjqdh", "48nine7sixfive", "22x", "sixrgtwo3rnbzkrztkdkg", "4t", "29bjpskmxneightppvthree", "zmlzxvtlkt4seveneightbxseven", "5two5eightnpszzmbkncnstx4", "9vk98sevenhznkxmlrlk7vdbqgvfjdk", "1sixb8sjkvdhfld", "one42eight4mrsdnpfjpvdtq", "76fourntsrfllxkdfqvm6seven", "skqndhr3nm4776", "4xpmfxmvj633eight", "83ninecmpt", "fourdthree9", "9eightjqnnmthcrseven", "7threekgtf1", "xscj7threenmhsixseven5s3", "cqlzjt41", "855threemlmmqkgtfk", "ninefzmvjjtvbmgf8nineninetwonegcn", "ccpkzcldfourkdtfkjxvfb9fourhbtwonsoneightnl", "pkeightwo5seven88rdnzzsdkbjeight9", "threen2fjsfivesix26nine", "nine4rz8nine7bglpcmkqfzpseven", "eight94six8dpgrv", "twodfctf278", "fltqtmdkgjsvf72three", "llrtzsixsix4fivetwosixone", "qjhtjqjhgkjkzlpxxclsrdnzk1gbqt", "sixeight1sixtwo", "one5413nkmqjtlbdkz22", "bhtwoneonemzpzkqeighttwooneqkmcmsbq4", "sevensix3three2sixprcqcvm", "25tjffdrtwohfqlkhzxlhb", "97gcgqgjnpsthfjfdv636jsxq", "zggjmjone1297six8drzs", "jbpvnineeightntkkshbjvr3nshnqzdlkjmkfive", "5four2gkkbxmpthreefour6", "5two15sixfivetzpg", "one4fouronemfpvnqseven", "9fnlbljdnzzfournine78", "djfljccrtvvqktzzvk61onesd", "7twohbkeight", "seven1eighttwothreet", "4mdcljknhpqgxffqpj5", "nine9jlsmfgdgntwothreeeight4", "136nh", "635ninejghg5", "cmone7fdlk9lfivemzvnhkcsp", "8eightnlndm", "6fourpb892", "fiveseventwosixfourthree7", "5fm", "ninegchdnrf63431", "24sgnflnsixninenine8", "snm9", "3fntd721dhhkrqqxsfpstsvzpgonetkhcr", "jlzfbml61vdmgb7one", "266517", "7fivetwo2vhchmg678nine", "cgrp3vzn5ninetwofour", "666ninefour", "9s", "svpcnlktpxtvk42jhsvvdpftxpsk", "2qznfzvbdr", "foneb7eightfivehlbjjknninethree", "kfp6", "l34pxxhxtd7d", "rsbcrtwo27twocqlmeight", "jkzgvqgpjfdqvmjfx2flnvjmgllxghhrbjjkfour2", "45sevengdnf59twofive", "6fivespvkblrxvkcgdxktl", "three9dvrssvl5eight4ftsix", "seven56gdmlbfbjsl894sevencmc", "814", "1one4", "onenine5fivekcrf1gvvfhlncsv", "2ctvq9djzddfxcrj", "ntdlcqgsixvmfvlc4fourvlhtvvqmnmkrm", "9nineseven1seven", "lcvzbnfourksvjqvmv47one5", "nine4blvlvlpkl6", "sixnqxrhnztzvpmbzmxjm19five", "18jtzhk", "rzrhv8four", "2npghxvjonebchsprfhsjznrxvxnine", "eightngsevencrjkxbhpgtxlzhgb46sevenqhqmlfx", "threesffl9fivelgmndjfvseven92", "seven85", "87six9vnshclz", "threetwo7915three", "one2vkbp6rhqbxvcl7", "bsbr1five91", "qd3mnine", "jjvhltxtdh5nineone6", "mbxlnj7bbhnxonejtmtqjfrzqgtrhkeightnine", "fourfourqrxdtfive2smnqp", "7tvjrszvrhdl5five", "four15tvmpvxpvdjnine", "sevenvv5tworpvdlseven3dlqvgblqtwo", "nkckggninegnlqlnv25threexlhlbzvzk", "3vngmhprjseventhreeeightnine", "nvqtpzsszrdvttfivenine56oneseven8", "146", "fxfbone59", "f32dhffctkxp6rcngvtfq", "sixthreefsixjhckmjqfive495", "42four", "65nine984", "5fthreeone9twoqqsfvzmp", "ttwonefive4", "one6gfxseightxqcq6", "3sixnrjtwormrncmhxeight", "jhdxnmsgsdsevensqsslbsndpdmznmldbgeight3tcvjjv4", "5sixtvpckxzcjzbmrzk9", "pmdmnfgkb3six8xsmstsmxgmm", "53onetvlgbglq4zbqpdgsskzdsksd6", "kzjcllvz6skphkfdxfiveqrbhmk", "75qqjdgxlmfthreevzbfjdlxkfqqq", "seveneightjntpjthzptwo2two", "2five4fvrfxxnine4qzkkfkmq", "2xlvcltn7", "fnmggtj2rqxzh7three", "rzpjkgtml1", "2oneseven4one7xps6", "rljfhfrhmzkjxktnszbkpfspxdkqneight2", "pzgnine49six2", "plxsqeight2", "eight2sevenseveneight8rfcrsdlxb", "sevenclpqqfxgjnmtwo9", "9sevenrqsixone8eightrxqgfsbjh", "kqtkstrxhtfzbllhl4lqvqkcbr", "hfplfpbltczflpp7nfive8", "ninenvqfrvtwo6onel", "threev65", "frhn18six9sixninefourrsqzgd", "mcxckfg5vpkbs89gbninexjzvlj", "fivesixdx28", "7ppbqv", "hs9twopcvpgtjnrsvksskpc8", "9mlpckzj2twothreefive", "rkrgdclkninetwo6eighttwodc25", "tfivefourtwohkhhgsqlj1dtdcxmxkf", "1four6five", "fgbvmvxvtsix2twonine2sixfour", "foureight66", "s6fourcv", "mxl358sixfive8six8", "ztbtwo73sixvxsix9four", "eight7qmdlcxfive5", "phgfivekrjxdmnzsqsix9", "1mfqsevenhz", "rjhcdgzngtc155bqlttbsxklpknvlmk", "qjkdqlrrs6two", "sxlmqzxdpxdnj9fivetwo9seven5", "2qtdblb2", "8qgdzrsixtwo598oneightp", "1shdb944", "vrlpronek2", "jm52", "8eightfourseven11mvtrmtkr2bmp", "mnvnjxrgmrxhztwo2ssrdpqk", "ztfive435three6threetwo", "tnrrdnbgnbhzljdxhxxfrqkcpeight8js3", "foursix6zcsrztvgjxmp", "five7fourgnnkspxcmczcbgsbdf77five", "fgbrzkmvgrdbqjqndpfive81onetwomtzlfb", "2qbsfd1two3ninetwo2", "8tdjxvfpvdvone33three", "lpchnmln56twofive8tfour", "cfkfbhppjf6fourdkfxsvdtbcjspzlseven8", "5fivestgkzsevenonedkhhrkthree", "37nine8six8onefhvvbkmgdfgtv", "26hzz", "5glvnsztmnfjmkjseventdm4five", "pvnnqrqvftrbcvnnthreenine5", "mgscxxlp3eight", "53eighteight", "two1oneqlcdkbddfour", "jbll3", "8threeseven5tmtrgdhqxd", "8twonine6s1", "91seven5pmqrjlhqrtzs", "jj3sevensix4482", "jeightwo7lk4three", "zchchxmsctzffivefournine9sqhqkgfour", "72xct1", "vnsxvsqkhpfvgdseven23gzcmltzgone", "xzjqhcvsix1fivecjtxnfivekmvjdc", "zdfourgjlhtwo24d5klkpdgqbz", "7sdzzdbrxbtonerjcmknnql4dfzqccvqt", "tncqzxjq9twofiveqkxdrxrpj894six", "dddmkctrzlpfmsszeight8zvbpmpkg", "three23ckjhgjc", "375jzdhnfcfr19mhsbnplqh", "vpbbjlzone5sevenseven33four", "onejzfsevenrbskjq1four", "seven13one", "vcnkfgv979one6zln", "rqlxzzbmjb4lmbthreektqsdcfzbmdsfivethreenrxdlkqt", "qkoneight8", "5rfourfivenine94fdprsix", "onexonelzdh2lcbqpzq6", "six6v", "7gtgxqnnine", "tsljzhntwo3fourpbjncgmvf3fflvjxp", "vfkdone9fivecftvmjdk", "xc5three6eight94", "18363one7", "8fiveksshdlfmzhljhcmjrn7kpv5j", "xbhmxfhbjnjzmninethree7", "2933mkmdqjcl", "6ncvzqxfvgfive", "lnine5fivetb4qmfktnqjxs", "93187", "5mqninedzkfhbk", "two7eightntdbsix298four", "sixone3bspxqxggkmkrbcqrhfrxrlgjrlvfl96", "fourfivehqls3nine", "threedfklszn2threeqzhh7one", "mqmftzglone6kjpgglznhrjz89", "146cvkftscqsevensixnine", "nndhdgpd484hxdgjtfsdxxg9", "6mbzckbjphg", "eight6jbjtnld2mdjtd", "zjtzcqxb736five", "jlkdmone8", "gvjnjvmlfvcmvnfb8xcgjcmjqvz1bzcctvsixfzqjlhfkfk6", "vr6onejnjmrrldnsixsix5six", "ninembtmtkgbctlfive45cjzzrmgcscfbcgeight", "2mdvneightjzgffivefive4", "hmdnbxghxjxt4czshmsfzc", "61six18threehrcj", "six3five6eightkdfzhxcjkdhq3", "jrhqrqkpd4hsixdsbjdpscclmnnhknqq16", "jflzcxr3three", "threefourghvgsktkc93cmjmsgh8one6", "96fivesevenslklhsfmpz", "jgkpgfnnbq2pmspdfhsqxfour", "g4fourthreerpkdhjhlxlzvnineseven", "xkxhkphnkvpdnlncn86srxthree", "7sixsevenrfour", "5zr72qltsrbdsv", "ninervqzdfzqmf6five", "8jslpvs73", "ztvlxndlm5twohdhmtrdnhbzdrxb", "seven6nine4dpdpvrtrmqvql", "jfz1", "5nineeight5onefivecxtqbsdtbthreefour", "fourgeight6threeszgseventwo9", "sixfour3", "npl8", "tzjkffsvbjseven5rhmlxonezlx", "5dhtpfour", "twothreebxtfndvdnine1sixbb9", "five9nineqlzrmtgs5", "9v764nineeight", "five4eightlsix6", "3nineeight21", "foureight8btsc", "3xgdgtb2", "7threetwonexqk", "kkqsix48onefourhlsh8", "onekgtdzgfh2fivenine2onerb", "six4zgcnlhmltrxp5xphvtwo9", "eight7cdqggpssix", "niner9pzmrbqldkljmgphrrgmdjseven6", "439", "twofoursixrthree5bxppnhqtx", "bmpnt3", "fivepkzkzpghrptpksevenseven83two1", "9fiveone8one", "fiveseven3lqxghdlskbltrzrstwo", "fournine3ninephlghonetwoeightbvmdcconeightq", "three2pvklmzqjfh4sixonedrctlsfdfour", "three91spjlscscjcxbbpdhrg37", "57qqjpdfppsix1qxrh5mlmncf", "4nfone5eight", "eightqsix7one", "4jtvxfd38hnrmqkbnvfxpp", "qmfsspkfour1plmslcrsseventhree", "fzckcbfvxbpsix7nine", "fzrj4", "4threeqntnineqstzjftnine", "tkrh6sixdqflrvtmzmfiveseven9ktmtvprkxhfour", "nine4983four", "mpllmjrfgv66five3kvhthplrtwo7nkklb", "9ngvdjddqbz", "5twosix8lbhmzrg", "eightsbmcfgm76two4hhc6", "seventwosevenrpm6threeeightwodxs", "xkbseventwotwogmkxhpmhm42hvvbfchreight", "gcqeightwosix8xdlhrnnbkmsevenqdbrjghz", "458ninextfjxvgsq5fltdsk6", "rlgsflhxqd5bdbhclmrthree", "twothreemqqbzjn88blvqxbseven", "rqrrdrmlfsixfive6", "eight959tzxkgqjd", "txdszrn5eight3cqeight1brqr", "45122", "jvvslnkdk6qnfzjzvseight55eight", "4twoeightgrhhkrvtkrzpfive7seven", "three8gsmkpzsmfvf2", "fiveeight5sevenone9twoseven", "4seightjjdkdglspz3vg", "sevenssrzkspld2", "qnzcvcthrsgjlnzxmxlppjdpnine8seven7", "eight7xhvkrcr", "two2tdjdfbqtqxrs119r"]
  in  "delimited string":string="ninefourone1\n53sevenvvqm\nkscpjfdxp895foureightckjjl1\n72fivebt9ndgq\n28gtbkszmrtmnineoneightmx\nfour66jqrbtqcsxjtqjvfjhl1\nfour8pzznjbhxlhtz6bhtzdxjlg1\nrgxjrsldrfmzq25szhbldzqhrhbjpkbjlsevenseven\nslkjvk4threesevenznjqmmfive\n61ppgrkmkfhteightone\n1threesix67px\nsxbjdbtlnjrmlzgxneightthreepmqxdxhfk8jfrheightwovp\ntwofour2sevenk\nsevenonezknqnkfqbzffjvfivetwo94two\n45xj\nmp7one6eightvhfnmfive6\nfhtctftxm3threefour2b\n2dq7bdmhhs92\npdnbqlbvtcxgpnfhmsfhzstgm173\n8fourvxkddsrlcvseveneight\n15zqpmsix77hlljgfive\njzjv6seven\neight1vbfive\n721sixsdzbqtskbpkqbcmgmlpk5psrhr\npqxdxcx5\ntwozsf2five\n7twosixthree775\n7xtxrch7six..."
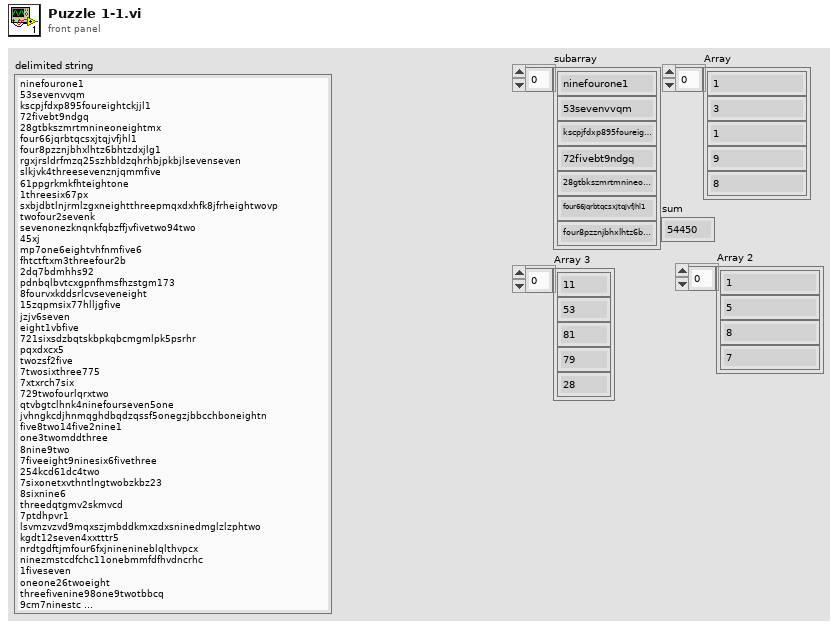
[diagram p1: front panel]
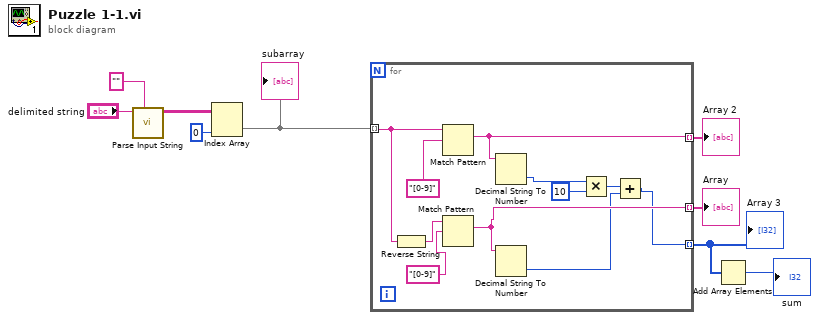
[diagram p0: block diagram]
diagram:
  n1 = call "Parse Input String.vi"("delimiter (Tab)"="", "delimited string"="delimited string") -> ("parsed string"=w7:string[][])  [unwired: 9 in]
  n2 = Index Array(array=w7, index (col)=0 ("disabled index (col)")) -> (element=w5:string[])  [unwired: 1 in]
  "subarray" <- w5
  n3 = for {
    tunnel: w5 -> [w19] mode=indexing
    tunnel: [w16] -> w4 mode=indexing
    tunnel: [w15] -> w3 mode=indexing
    tunnel: [w10] -> w2 mode=indexing
    n4 = Reverse String(1:w19) -> (0:w17:string)
    n5 = Match Pattern(string=w19, regular expression="[0-9]" ("format string")) -> (match substring=w16:string)  [unwired: 1 in, 3 out]
    n6 = Match Pattern(string=w17, regular expression="[0-9]" ("format string")) -> (match substring=w15:string)  [unwired: 1 in, 3 out]
    n7 = Decimal String To Number(string=w16) -> (number=w14:i32)  [unwired: 2 in, 1 out]
    n8 = Decimal String To Number(string=w15) -> (number=w11:i32)  [unwired: 2 in, 1 out]
    n9 = Multiply(x=w14, y=10) -> (x*y=w12:i32)
    n10 = Add(x=w12, y=w11) -> (x+y=w10:i32)
  }
  "Array" <- w3
  "Array 2" <- w4
  "Array 3" <- w2
  n11 = Add Array Elements(numeric array=w2) -> (sum=→"sum":i32)
